vi "target menu name.vi"(8 "error in":errorcluster, 11 "PLTarget PXI in":refnum<class "PLTarget PXI.lvclass">) -> (0 "error out":errorcluster, 2 "menu name":string, 3 "PLTarget PXI out":refnum<class "PLTarget PXI.lvclass">)   [LabVIEW 2013, in "PLTarget PXI.lvclass"]
uses:
  PLTarget PXI.lvclass
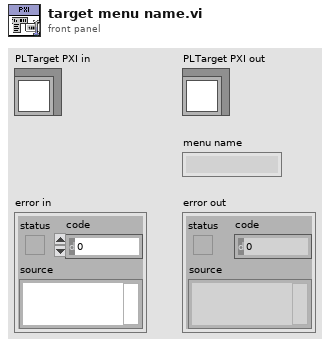
[diagram p1: front panel]
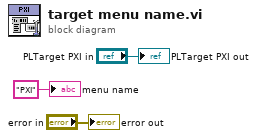
[diagram p0: block diagram]
diagram:
  "error out" <- "error in"
  "PLTarget PXI out" <- "PLTarget PXI in"
  "menu name" <- "PXI" ("menu name")
